vi "9.1.vi"() -> ()   [LabVIEW 2019]
panel:
  out "C":bool
  out "E":bool
  out "F":bool
  out "B":bool
  out "D":bool
  out "G":bool
  out "A":bool
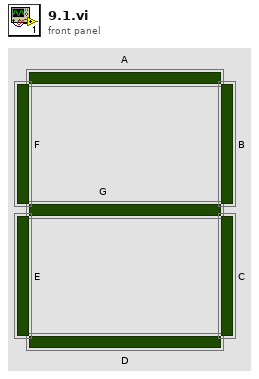
[diagram p1: front panel]
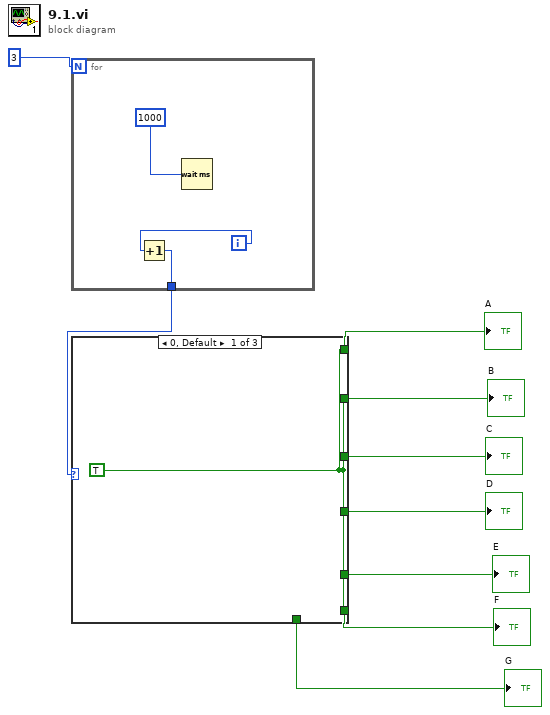
[diagram p0: block diagram]
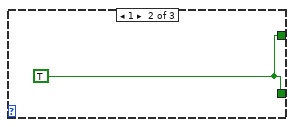
[diagram p2: hidden frame]
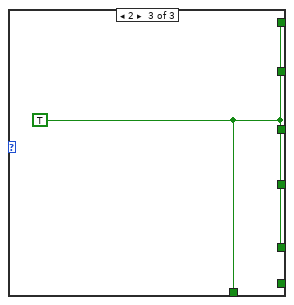
[diagram p3: hidden frame]
diagram:
  n1 = for {
    N: 3 -> [_]
    tunnel: [w10] -> w1
    i -> [w11]
    n2 = Increment(x=w11) -> (x+1=w10:i32)
    n3 = Wait (ms)(milliseconds to wait=1000) -> ()  [unwired: 1 out]
  }
  n4 = case shown="0, Default" w1 {
    tunnel: [w13 _ w15] -> w9
    tunnel: [w13 w14 w15] -> w8
    tunnel: [w13 w14 _] -> w7
    tunnel: [w13 _ w15] -> w6
    tunnel: [w13 _ w15] -> w5
    tunnel: [w13 _ _] -> w4
    tunnel: [_ _ w15] -> w3
    frame 0, Default {
      w13 = TRUE
    }
    frame 1 {
      w14 = TRUE
    }
    frame 2 {
      w15 = TRUE
    }
  }
  "G" <- w3
  "A" <- w9
  "B" <- w8
  "C" <- w7
  "D" <- w6
  "E" <- w5
  "F" <- w4
